vi "VISA POLL.vi"(8 "Error In":errorcluster, 9 "Test Duration (ms)":u32=10000, 10 "Loop Delay (ms)":u32=100, 11 "VISA resource":refnum<visa-resource-name>="COM3") -> (0 "Error Out":errorcluster, 1 "Instrument Data(Random)":string, 3 "Correct Response Rate %":dbl(slide) scale=0.0..100.0, 4 "No of Reponse":i32, 5 "False Polling":i32)   [LabVIEW 2015]
uses:
  <vilib>/Instr/_visa.llb/VISA Configure Serial Port (Instr).vi
panel:
  in  "STOP":bool
  # "Polling"
  # "x 100"
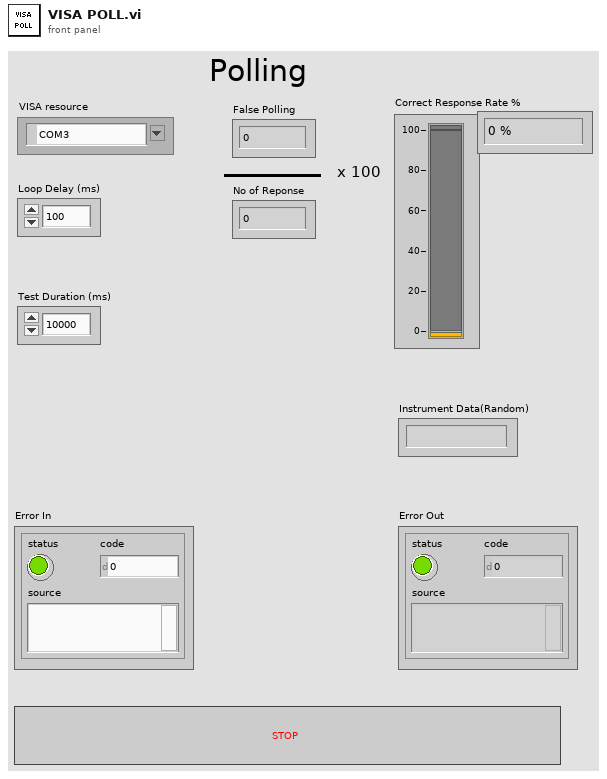
[diagram p1: front panel]
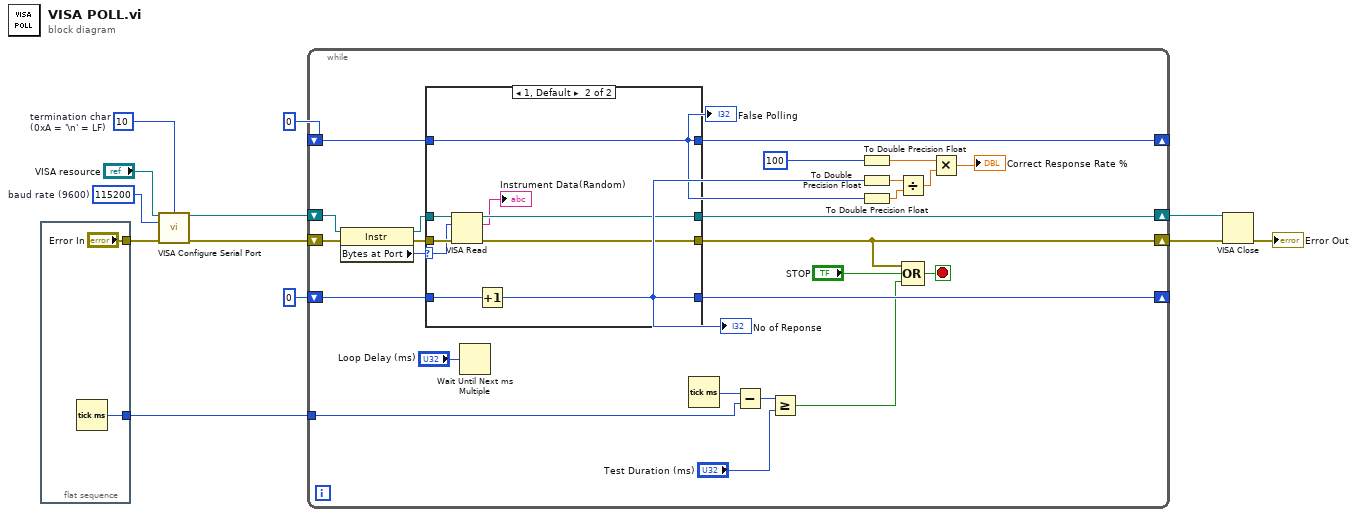
[diagram p0: block diagram]
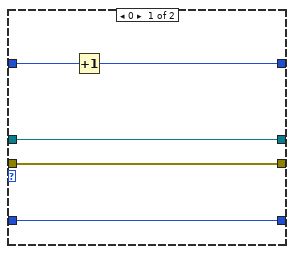
[diagram p2: hidden frame]
diagram:
  w11 = u8 10  # termination char (0xA = '\n' = LF)
  w12 = u32 115200  # baud rate (9600)
  n1 = flat-sequence {
    tunnel: ["Error In"] -> w9
    tunnel: [w13] -> w2
    frame #0 {
      n2 = Tick Count (ms)() -> (millisecond timer value=w13:u32)
    }
  }
  n3 = call-poly "VISA Configure Serial Port"("VISA resource name"="VISA resource", "termination char\n(0xA = '\\n' = LF)"=w11, "baud rate (9600)"=w12, "error in (no error)"=w9) -> ("VISA resource name out"=w4:refnum<visa-resource-name>, "error out"=w3:errorcluster)  [unwired: 10 in]
  n4 = while {
    shift-right: [w24] -> _
    shift-left: 0 -> [w31]
    shift-right: [w25] -> _
    shift-left: 0 -> [w29]
    shift-right: [w33] -> w6
    shift-left: w3 -> [w37]
    shift-right: [w32] -> w5
    shift-left: w4 -> [w38]
    tunnel: w2 -> [w17]
    stop <- w30 stop-if-true
    n5 = property class="Instr"(reference=w38, error in=w37) -> (reference out=w35:refnum<visa-resource-name>, error out=w36:errorcluster, "Bytes at Port"=w34:u32)
    n6 = case shown="1, Default" w34 {
      selector: w34 -> [_ w49]
      tunnel: w36 -> [w43 w53]
      tunnel: [w43 w52] -> w33
      tunnel: w35 -> [w44 w51]
      tunnel: [w44 w50] -> w32
      tunnel: w31 -> [w42 w47]
      tunnel: [w41 w47] -> w24
      tunnel: w29 -> [w40 w46]
      tunnel: [w40 w45] -> w25
      frame 0 {
        n7 = Increment(x=w42) -> (x+1=w41:i32)
      }
      frame 1, Default {
        n8 = VISA Read(VISA resource name=w51, byte count=w49, error in (no error)=w53) -> (VISA resource name out=w50:refnum<visa-resource-name>, read buffer=→"Instrument Data(Random)":string, error out=w52:errorcluster)  [unwired: 1 out]
        n9 = Increment(x=w46) -> (x+1=w45:i32)
      }
    }
    "False Polling" <- w24
    "No of Reponse" <- w25
    n10 = Wait Until Next ms Multiple(millisecond multiple="Loop Delay (ms)") -> ()  [unwired: 1 out]
    n11 = Tick Count (ms)() -> (millisecond timer value=w18:u32)
    n12 = Subtract(x=w18, y=w17) -> (x-y=w19:u32)
    n13 = Greater Or Equal?(x=w19, y="Test Duration (ms)") -> (x >= y?=w16:bool)
    n14 = To Double Precision Float(number=100 ("x")) -> (double precision float=w22:dbl)
    n15 = To Double Precision Float(number=w25) -> (double precision float=w27:dbl)
    n16 = To Double Precision Float(number=w24) -> (double precision float=w26:dbl)
    n17 = Divide(x=w27, y=w26) -> (x/y=w21:dbl)
    n18 = Compound Arithmetic op=OR(w33, "STOP", w16) -> (w30:bool)
    n19 = Multiply(x=w22, y=w21) -> (x*y=→"Correct Response Rate %":dbl)
  }
  n20 = VISA Close(VISA resource name=w5, error in (no error)=w6) -> (error out=→"Error Out":errorcluster)
